vi "Set Columns.vi"(3 "error in (no error)":errorcluster, 4 "Columns":refnum<class "Column.lvclass">[](array[class]), 5 "Arduino DDS in":refnum<class "Arduino DDS.lvclass">) -> (0 "error out":errorcluster, 1 "Arduino DDS out":refnum<class "Arduino DDS.lvclass">)   [LabVIEW 2013, in "Arduino DDS.lvclass"]
uses:
  Arduino DDS.lvclass
  ColumnVIs/Column/Column.lvclass
  Device/Device.lvclass
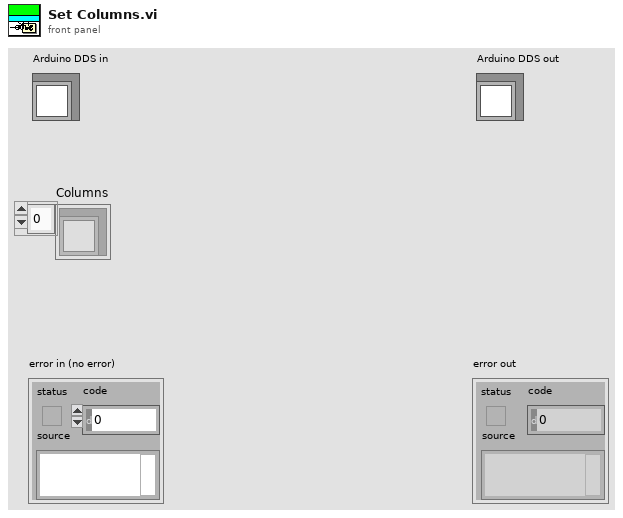
[diagram p1: front panel]
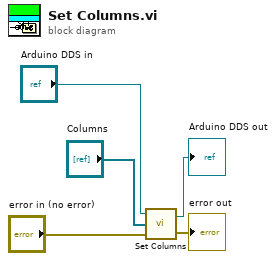
[diagram p0: block diagram]
diagram:
  n1 = call-parent "Set Columns.vi"("error in (no error)"="error in (no error)", "Columns"="Columns", "Device in"="Arduino DDS in") -> ("error out"=→"error out":errorcluster, "Device out"=→"Arduino DDS out":refnum<class "Arduino DDS.lvclass">)  [unwired: 1 in]
